vi "PSK_Mod_Receive_logger.vi"() -> ()   [LabVIEW 2014]
uses:
  <vilib>/addons/Modulation/Digital/General/MT Generate Bits (Galois, PN Order).vi
  <vilib>/addons/Modulation/Digital/Support/Common/Validators/mod_Generate Bits Validate.vi
  <vilib>/addons/Modulation/Analog/support/mod_Set Error Source.vi
  <vilib>/addons/Modulation/Digital/General/MT Generate PSK System Parameters(M).vi
  <vilib>/addons/Modulation/Digital/Support/Common/Validators/mod_Generate Filter Coefficients Validate.vi
  <vilib>/addons/Modulation/Digital/General/subVIs/mod_Generate Filter Coefficients.vi
  <vilib>/addons/Modulation/Digital/General/subVIs/mod_Generate Bits PN Sequence.vi
  <vilib>/addons/Modulation/Digital/General/MT Generate PSK Synchronization Parameters (bit array).vi
  <instrlib>/niUSRP/niUSRP Fetch Rx Data (CDB Cluster).vi
  <vilib>/Utility/file.llb/Write To Spreadsheet File (I64).vi
  <vilib>/addons/Modulation/niDMT.lvlib
  <vilib>/addons/Modulation/niAMT.lvlib
panel:
  out "Before demod&compensation":waveform(dbl)(graph)
  out "Constellation Graph":T1(graph) caption="Rx Signal Constellation"
  out "sync found index (symbols)":dbl format="%.4f"
  out "Bits received":i32
  in  "Guard bits":i32=20
  out "Demod loop time":dbl
  out "USRP loop time":dbl
  in  "Header bits":i32=16
  in  "stop":bool
  out "bits received":i32
  out "Aquisition time":dbl
  in  "Message bits":i32=128
  in  "Sync bits":i32=30
  out "sync correct?":bool
  out "output bit stream":i8[](array[numeric])
  out "error out":errorcluster={"status"=FALSE, "code"=1074118647, "source"="niUSRP Fetch Rx Data (CDB Cluster).vi<ERR>Overflow: an internal receive buffer has filled before the data could be returned.  Consider reducing the IQ rate, increasing the Fetch rate, or increasing the number of samples per Fetch."}
  in  "USRP IP Address":refnum<k15>="192.168.10.1"
  out "Actual Rx Parameters":T2={"Rx IQ Sampling\nRate [s/sec]"=200000.0, "Rx\nFrequency [Hz]"=915000000.0, "Rx Gain [dB]"=20.0, "Rx Antenna"="RX1"} {"Rx Gain [dB]" format="%#.6p"; "Rx\nFrequency [Hz]" format="%#.6p"; "Rx IQ Sampling\nRate [s/sec]" format="%#.6p"}
  in  "Rx Parameters":T2={"Rx IQ Sampling\nRate [s/sec]"=400000.0, "Rx\nFrequency [Hz]"=5795000000.0, "Rx Gain [dB]"=0.0, "Rx Antenna"="RX1"} {"Rx Gain [dB]" format="%#.6p"; "Rx\nFrequency [Hz]" format="%#.6p"; "Rx IQ Sampling\nRate [s/sec]" format="%#.6p"}
  in  "Packets per burst":i32=20
  in  "filter parameters":T3={"Alpha"=0.5, "Filter Length"=6, "TX Filter"=enum."Root Raised Cos"} {"Alpha" format="%.2f"}
  in  "QPSK System Parameters":T4={"Samples per Symbol"=8, "symbol map"=[], "Differential PSK"=enum."disable", "PSK type"=0} {"PSK type" items=["normal", "shifted", "offset"]; "symbol map" format="%.3f"}
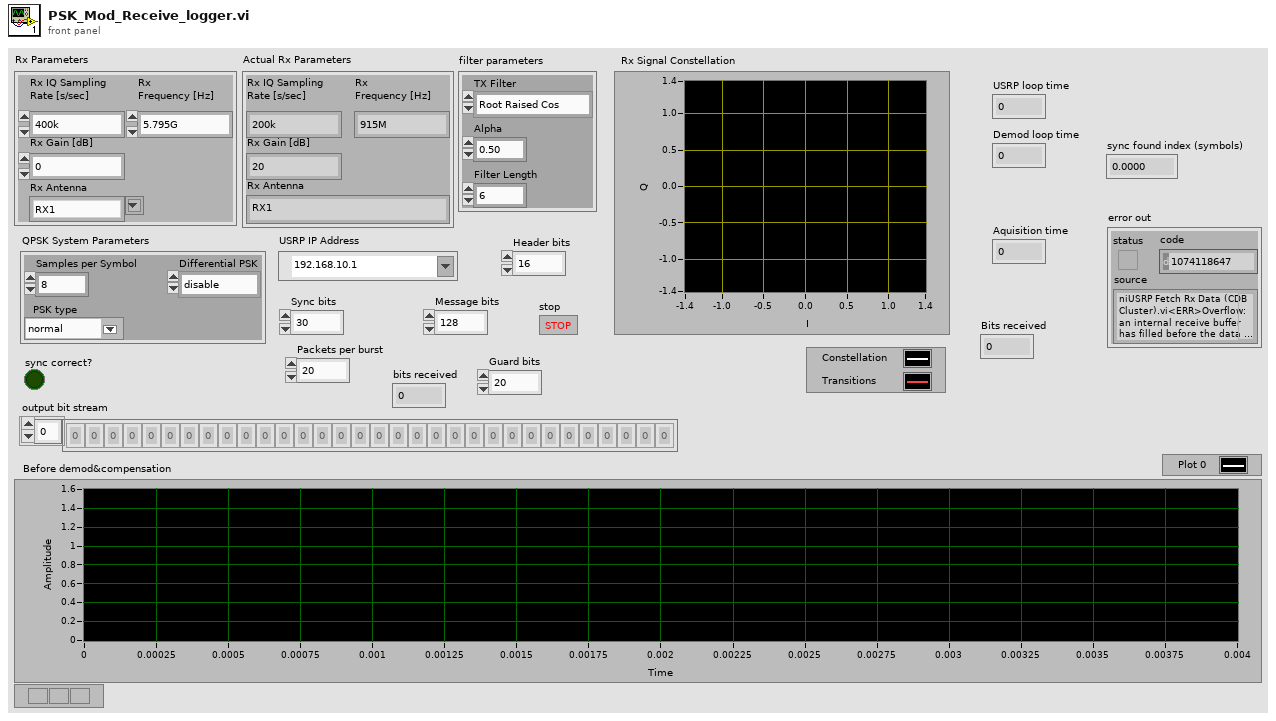
[diagram p1: front panel]
types:
  T1 = cluster{"constellation":dbl[], "oversampled data":dbl[]}[]
  T2 = cluster{"Rx IQ Sampling\nRate [s/sec]":dbl, "Rx\nFrequency [Hz]":dbl, "Rx Gain [dB]":dbl, "Rx Antenna":string}
  T3 = cluster{"Alpha":dbl, "Filter Length":i32, "TX Filter":enum16{"none", "Raised Cosine", "Root Raised Cos", "Gaussian"}}
  T4 = cluster{"Samples per Symbol":i32, "symbol map":cdb[], "Differential PSK":enum16{"disable", "enable"}, "PSK type":u16}
  T5 = enum16{"FSK", "PSK", "QAM", "MSK", "PAM", "ASK", "CPM"}
  T6 = enum16{"none", "Raised Cosine", "Root Raised Cos", "Gaussian"}
  T7 = cluster{"samples per symbol (16)":i32, "symbol map":cdb[], "differential PSK":enum16{"disable", "enable"}, "PSK type":u16}
  T8 = cluster{"expected sync location (symbols)":i32, "sync sequence":cdb[], "sync location uncertainty (symbols)":i32, "sync indent (symbols)":i32}
  T9 = typedef "niAMT.lvlib/Complex Data Waveform.ctl" = cluster{"t0":dbl, "dt":dbl, "Y":cdb[]}
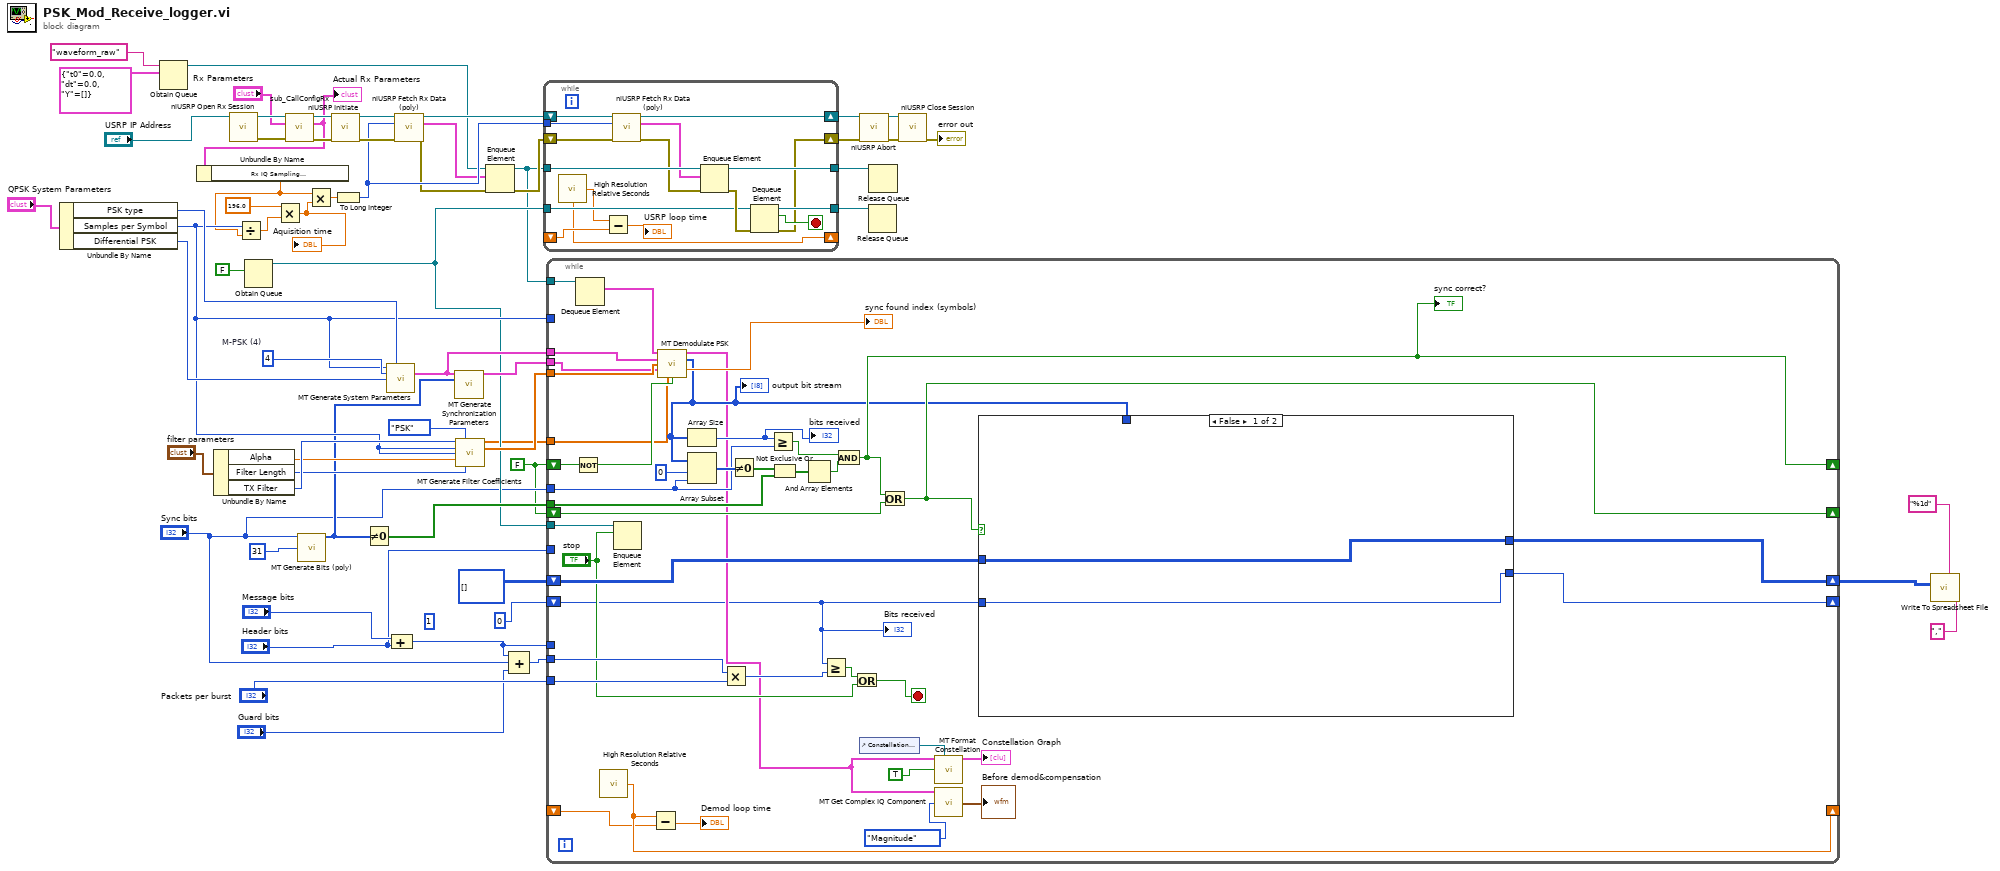
[diagram p0: block diagram]
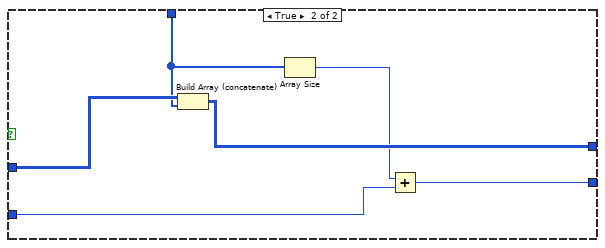
[diagram p2: hidden frame]
diagram:
  w7 = FALSE
  (unwired) 1 ("dimension size")
  w60 = 4  # M-PSK (4)
  n1 = Unbundle By Name("QPSK System Parameters") -> ("PSK type"=w35:u16, "Samples per Symbol"=w32:i32, "Differential PSK"=w61:enum16{"disable", "enable"})
  n2 = Obtain Queue(name (unnamed)="waveform_raw", element data type=cluster{"t0":dbl, "dt":dbl, "Y":cdb[]} {"t0"=0.0, "dt"=0.0, "Y"=[]} ("data")) -> (queue out=w27:refnum<queue>)  [unwired: 3 in, 2 out]
  n3 = Unbundle By Name("filter parameters") -> ("Alpha"=w57:dbl, "Filter Length"=w58:i32, "TX Filter"=w59:T6)
  n4 = call <instrlib>:"niUSRP Open Rx Session.vi"("device names"="USRP IP Address") -> ("session handle out"=w51:refnum<k15>, "error out"=w52:errorcluster)  [unwired: 13 in]
  n5 = Obtain Queue(element data type=FALSE) -> (queue out=w17:refnum<queue>)  [unwired: 4 in, 2 out]
  n6 = call "sub_CallConfigRx.vi"("session handle"=w51, "Rx Parameters"="Rx Parameters", "error in"=w52) -> ("session handle out"=w49:refnum<k15>, "Actual Rx Parameters"=w46:T2, "error out"=w48:errorcluster)  [unwired: 10 in]
  "Actual Rx Parameters" <- w46
  n7 = Unbundle By Name(w46) -> ("Rx IQ Sampling\nRate [s/sec]"=w23:dbl)
  n8 = Divide(x=w32, y=w23) -> (x/y=w30:dbl)
  n9 = Multiply(x=196.0, y=w30) -> (x*y=w11:dbl)
  "Aquisition time" <- w11
  n10 = call-poly <vilib>:"MT Generate Bits (poly).vi"("total bits (128)"="Sync bits", "PN sequence order (9)"=31) -> ("output bit stream"=w19:i8[])  [unwired: 11 in, 2 out]
  n11 = Multiply(x=w23, y=w11) -> (x*y=w53:dbl)
  n12 = call <instrlib>:"niUSRP Initiate.vi"("session handle"=w49, "error in (no error)"=w48) -> ("session handle out"=w45:refnum<k15>, "error out"=w44:errorcluster)  [unwired: 12 in]
  n13 = To Long Integer(number=w53) -> (32bit integer=w37:i32)
  n14 = Not Equal To 0?(x=w19) -> (x != 0?=w18:bool[])
  n15 = call-poly <vilib>:"MT Generate System Parameters.vi"("samples per symbol (16)"=w32, "PSK type"=w35, "M-PSK (4)"=w60, "differential PSK"=w61) -> ("PSK system parameters"=w34:T7)  [unwired: 9 in, 2 out]
  n16 = Compound Arithmetic op=ADD("Message bits", "Header bits") -> (w13:i32)
  n17 = call-poly <instrlib>:"niUSRP Fetch Rx Data (poly).vi"("session handle"=w45, "number of samples"=w37, "error in (no error)"=w44) -> ("session handle out"=w40:refnum<k15>, "data"=w25:cluster{"t0":dbl, "dt":dbl, "Y":cdb[]}, "error out"=w24:errorcluster)  [unwired: 9 in, 1 out]
  n18 = call-poly <vilib>:"MT Generate Synchronization Parameters.vi"("PSK system parameters"=w34, "sync bits"=w19) -> ("PSK synchronization parameters"=w33:T8)  [unwired: 12 in, 1 out]
  n19 = call <vilib>:"MT Generate Filter Coefficients.vi"("pulse shaping filter (none)"=w59, "modulation type"=T5."PSK", "pulse shaping samples per symbol (16)"=w32, "matched samples per symbol (16)"=w32, "filter parameter"=w57, "filter length (symbols)"=w58) -> ("pulse shaping filter coefficients"=w6:dbl[], "matched filter coefficients"=w36:dbl[])  [unwired: 7 in, 1 out]
  n20 = Enqueue Element(queue=w27, element=w25, error in (no error)=w24) -> (queue out=w1:refnum<queue>, error out=w26:errorcluster)  [unwired: 1 in, 1 out]
  n21 = Compound Arithmetic op=ADD(w13, "Sync bits", "Guard bits") -> (w14:i32)
  n22 = while {
    tunnel: w37 -> [w75]
    shift-right: [w77] -> w39
    shift-left: w40 -> [w78]
    shift-right: [w68] -> w38
    shift-left: w26 -> [w76]
    tunnel: w1 -> [w74]
    tunnel: [w71] -> w8
    tunnel: [w70] -> w21
    tunnel: w17 -> [w66]
    shift-right: [w64] -> _
    shift-left: _ -> [w65]
    stop <- w69 stop-if-true
    n23 = call <vilib>:"High Resolution Relative Seconds.vi"() -> ("relative seconds"=w64:dbl)
    n24 = Subtract(x=w64, y=w65) -> (x-y=→"USRP loop time":dbl)
    n25 = call-poly <instrlib>:"niUSRP Fetch Rx Data (poly).vi"("session handle"=w78, "number of samples"=w75, "error in (no error)"=w76) -> ("session handle out"=w77:refnum<k15>, "data"=w73:cluster{"t0":dbl, "dt":dbl, "Y":cdb[]}, "error out"=w72:errorcluster)  [unwired: 9 in, 1 out]
    n26 = Enqueue Element(queue=w74, element=w73, error in (no error)=w72) -> (queue out=w71:refnum<queue>, error out=w67:errorcluster)  [unwired: 1 in, 1 out]
    n27 = Dequeue Element(queue=w66, error in (no error)=w67) -> (queue out=w70:refnum<queue>, element=w69:bool, error out=w68:errorcluster)  [unwired: 1 in, 1 out]
  }
  n28 = while {
    tunnel: w36 -> [w93]
    tunnel: w34 -> [w94]
    tunnel: w33 -> [w92]
    tunnel: w32 -> [_]
    tunnel: "Sync bits" -> [w111]
    shift-right: [w98] -> _
    shift-left: w7 -> [w120]
    tunnel: w17 -> [w113]
    tunnel: w18 -> [w110]
    tunnel: w14 -> [w104]
    tunnel: w13 -> [_]
    shift-right: [w106] -> w4
    shift-left: i8[][] [] ("output bit stream 2") -> [w105]
    tunnel: "Header bits" -> [_]
    shift-right: [w109] -> _
    shift-left: _ -> [w108]
    tunnel: "Packets per burst" -> [w103]
    shift-right: [w96] -> _
    shift-left: w7 -> [w97]
    tunnel: w6 -> [w90]
    shift-right: [w81] -> _
    shift-left: i8 0 ("element") -> [w80]
    tunnel: w1 -> [w79]
    stop <- w102 stop-if-true
    n29 = Not(x=w120) -> (.not. x?=w91:bool)
    n30 = Dequeue Element(queue=w79) -> (element=w95:cluster{"t0":dbl, "dt":dbl, "Y":cdb[]})  [unwired: 2 in, 3 out]
    n31 = call <vilib>:"High Resolution Relative Seconds.vi"() -> ("relative seconds"=w109:dbl)
    n32 = Enqueue Element(queue=w113, element="stop") -> ()  [unwired: 2 in, 3 out]
    n33 = Subtract(x=w109, y=w108) -> (x-y=→"Demod loop time":dbl)
    n34 = call <vilib>:"MT Demodulate PSK.vi"("input complex waveform"=w95, "PSK system parameters"=w94, "matched filter coefficients"=w93, "synchronization parameters"=w92, "pulse shaping filter coefficients"=w90, "reset? (T)"=w91) -> ("recovered complex waveform"=w83:T9, "output bit stream"=w88:i8[], "sync found index (symbols)"=→"sync found index (symbols)":dbl)  [unwired: 5 in, 2 out]
    "output bit stream" <- w88
    n35 = Array Size(array=w88) -> (size(s)=w112:i32)
    "bits received" <- w112
    n36 = Array Subset(array=w88, index=0, length=w111) -> (w118:i8[])
    n37 = Multiply(x=w104, y=w103) -> (x*y=w99:i32)
    n38 = Not Equal To 0?(x=w118) -> (x != 0?=w116:bool[])
    n39 = Greater Or Equal?(x=w112, y=w111) -> (x >= y?=w115:bool)
    n40 = Not Exclusive Or(1:w110, 2:w116) -> (0:w117:bool[])
    n41 = And Array Elements(Boolean array=w117) -> (logical AND=w114:bool)
    n42 = Greater Or Equal?(x=w80, y=w99) -> (x >= y?=w100:bool)
    n43 = And(x=w115, y=w114) -> (x .and. y?=w98:bool)
    "sync correct?" <- w98
    n44 = Or(x=w100, y="stop") -> (x .or. y?=w102:bool)
    n45 = control-ref of="Constellation Graph"() -> (w87:refnum<vi>)
    n46 = Or(x=w98, y=w97) -> (x .or. y?=w96:bool)
    n47 = call <vilib>:"MT Format Constellation.vi"("waveform"=w83, "constellation reference"=w87, "autoscale"=TRUE) -> ("constellation graph"=→"Constellation Graph":T1)  [unwired: 11 in, 1 out]
    n48 = call <vilib>:"MT Get Complex IQ Component.vi"("IQ data (complex) in"=w83, "component choice"=enum16{"I", "Q", "Magnitude", "Phase"}."Magnitude") -> ("CE component"=→"Before demod&compensation":waveform(dbl))  [unwired: 11 in, 2 out]
    n49 = case shown="False" w96 {
      tunnel: w105 -> [w122 w127]
      tunnel: [w122 w128] -> w106
      tunnel: w88 -> [_ w126]
      tunnel: w80 -> [w121 w125]
      tunnel: [w121 w123] -> w81
      frame False {
      }
      frame True {
        n50 = Build Array (concatenate)(w127, w126) -> (w128:i8[][])
        n51 = Array Size(array=w126) -> (size(s)=w124:i32)
        n52 = Add(x=w124, y=w125) -> (x+y=w123:i32)
      }
    }
    "Bits received" <- w80
  }
  n53 = call <instrlib>:"niUSRP Abort.vi"("session handle"=w39, "error in (no error)"=w38) -> ("session handle out"=w42:refnum<k15>, "error out"=w43:errorcluster)  [unwired: 12 in]
  n54 = Release Queue(queue=w21) -> ()  [unwired: 2 in, 3 out]
  n55 = Release Queue(queue=w8) -> ()  [unwired: 2 in, 3 out]
  n56 = call <instrlib>:"niUSRP Close Session.vi"("session handle"=w42, "error in (no error)"=w43) -> ("error out"=→"error out":errorcluster)  [unwired: 13 in]
  n57 = call-poly <vilib>:"Write To Spreadsheet File.vi"("delimiter (\\t)"="," ("delimiter (\\t)"), "format (%d)"="%1d", "2D data"=w4) -> ()  [unwired: 5 in, 1 out]
